vi "Josephus_problem.vi"(8 "m":i32, 11 "N":i32) -> (2 "Last":dbl)   [LabVIEW 2019]
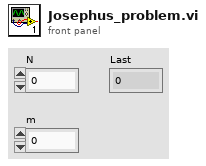
[diagram p1: front panel]
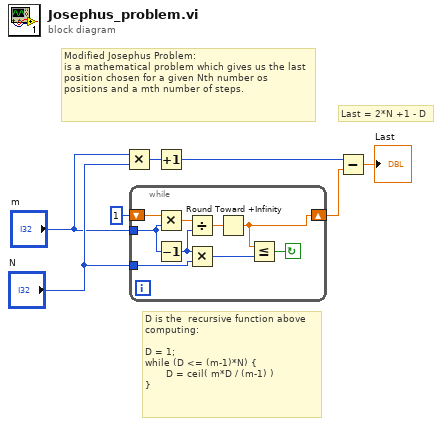
[diagram p0: block diagram]
diagram:
  # "Modified Josephus Problem:\nis a mathematical problem which gives us the last position chosen for a given Nth number os positions and a mth number of steps."
  # "D is the  recursive function above\ncomputing:\n\nD = 1;\nwhile (D <= (m-1)*N) {\n       D = ceil( m*D / (m-1) )\n}"
  # "Last = 2*N +1 - D"
  n1 = Multiply(x="m", y="N") -> (x*y=w5:i32)
  n2 = while {
    shift-right: [w10] -> w3
    shift-left: 1 -> [w15]
    tunnel: "N" -> [w11]
    tunnel: "m" -> [w13]
    stop <- w16 continue-if-true
    n3 = Multiply(x=w15, y=w13) -> (x*y=w14:dbl)
    n4 = Decrement(x=w13) -> (x-1=w8:i32)
    n5 = Divide(x=w14, y=w8) -> (x/y=w12:dbl)
    n6 = Multiply(x=w8, y=w11) -> (x*y=w9:i32)
    n7 = Round Toward +Infinity(x=w12) -> (ceil(x): smallest int >= x=w10:dbl)
    n8 = Less Or Equal?(x=w10, y=w9) -> (x <= y?=w16:bool)
  }
  n9 = Increment(x=w5) -> (x+1=w4:i32)
  n10 = Subtract(x=w4, y=w3) -> (x-y=→"Last":dbl)
